vi "Read_configuration.vi"(8 "error in (no error)":errorcluster, 11 "configuration file path":path) -> (0 "error out":errorcluster, 3 "output cluster":T1)   [LabVIEW 2015]
uses:
  <vilib>/LabVIEW Targets/FPGA/cRIO/shared/nicrio_ModuleControls/nicrio_cRIO-9234_DataRatesRing2.ctl
  <vilib>/Utility/config.llb/Read Key (Double).vi
  <vilib>/Utility/config.llb/Read Key (String).vi
  <vilib>/Utility/config.llb/Read Key (U32).vi
  <vilib>/Utility/config.llb/Read Key (Boolean).vi
  <vilib>/Utility/config.llb/NI_LVConfig.lvlib
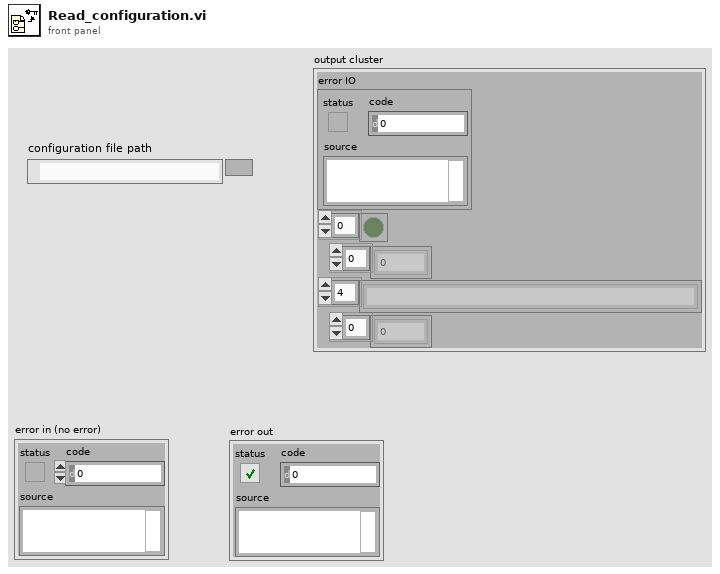
[diagram p1: front panel]
types:
  T1 = cluster{"error IO":errorcluster, bool[], u32[], string[], dbl[]}
  T2 = typedef "nicrio_cRIO-9234_DataRatesRing2.ctl" = u8
  T3 = typedef "NI_LVConfig.lvlib/Config Data RefNum.ctl" = refnum<k1>
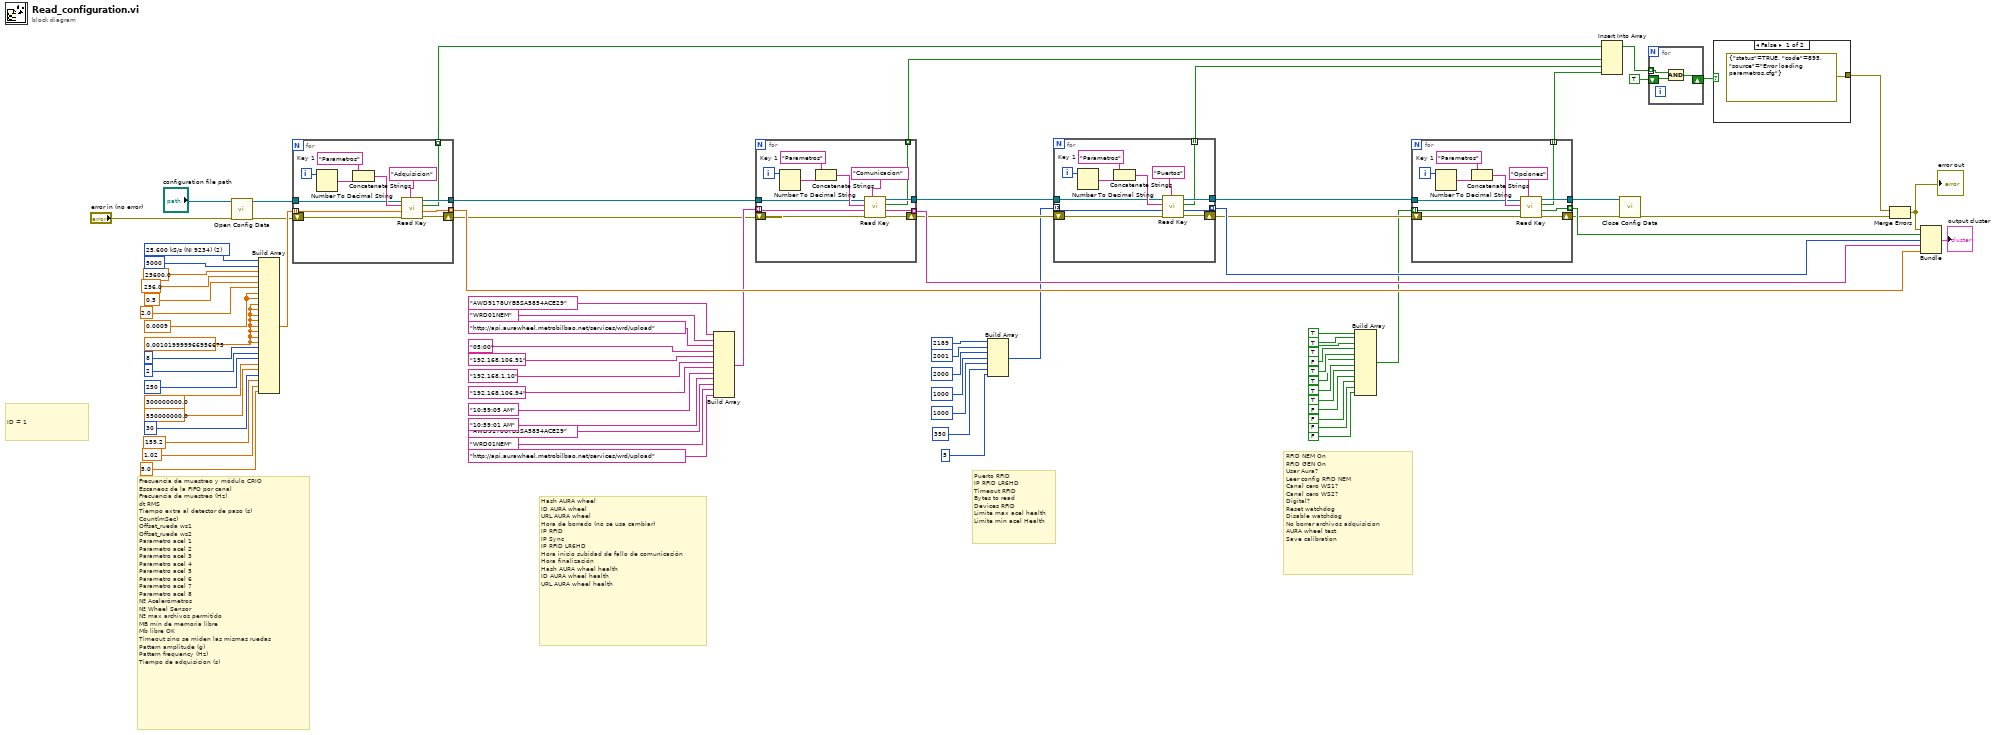
[diagram p0: block diagram]
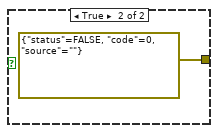
[diagram p2: hidden frame]
diagram:
  w34 = T2 2 items=["51.200 kS/s (NI 9234)"=1, "25.600 kS/s (NI 9234)"=2, "17.067 kS/s (NI 9234)"=3, "12.800 kS/s (NI 9234)"=4, "10.240 kS/s (NI 9234)"=5, "8.533 kS/s (NI 9234)"=6, "7.314 kS/s (NI 9234)"=7, "6.400 kS/s (NI 9234)"=8, "5.689 kS/s (NI 9234)"=9, "5.120 kS/s (NI 9234)"=10, "4.654 kS/s (NI 9234)"=11, "4.267 kS/s (NI 9234)"=12, "3.938 kS/s (NI 9234)"=13, "3.657 kS/s (NI 9234)"=14, "3.413 kS/s (NI 9234)"=15, "3.200 kS/s (NI 9234)"=16, "3.012 kS/s (NI 9234)"=17, "2.845 kS/s (NI 9234)"=18, "2.695 kS/s (NI 9234)"=19, "2.560 kS/s (NI 9234)"=20, "2.438 kS/s (NI 9234)"=21, "2.328 kS/s (NI 9234)"=22, "2.226 kS/s (NI 9234)"=23, "2.133 kS/s (NI 9234)"=24, "2.048 kS/s (NI 9234)"=25, "1.969 kS/s (NI 9234)"=26, "1.896 kS/s (NI 9234)"=27, "1.829 kS/s (NI 9234)"=28, "1.765 kS/s (NI 9234)"=29, "1.707 kS/s (NI 9234)"=30, "1.652 kS/s (NI 9234)"=31] ("Data Rate")
  w15 = 0.0009 ("element")
  w33 = sgl 0.00102
  # "RFID NEM On\nRFID GEN On\nUsar Aura?\nLeer config RFID NEM\nCanal cero WS1?\nCanal cero WS2?\nDigital?\nReset watchdog\nDisable watchdog\nNo borrar archivos adquisicion\nAURA wheel test\nSave calibration"
  # "Puerto RFID\nIP RFID LR6HD\nTimeout RFID\nBytes to read\nDevices RFID\nLimite max acel health\nLimite min acel Health"
  # "Hash AURA wheel\nID AURA wheel\nURL AURA wheel\nHora de borrado (no se usa cambiar)\nIP RFID\nIP Sync\nIP RFID LR6HD\nHora inicio subidad de fallo de comunicación\nHora finalización\nHash AURA wheel health\nID AURA wheel health\nURL AURA wheel health"
  # "Frecuencia de muestreo y módulo CRIO\nEscaneos de la FIFO por canal\nFrecuencia de muestreo (Hz)\ndt RMS\nTiempo extra al detector de paso (s)\nCount(mSec)\nOffset_rueda ws1\nOffset_rueda ws2\nParametro acel 1\nParametro acel 2\nParametro acel 3\nParametro acel 4\nParametro acel 5\nParametro acel 6\nParametro acel 7\nParametro acel 8\nNº Acelerómetros\nNº Wheel Sensor\nNº max archivos permitido\nMB mín de memoria libre\nMb libre OK\nTimeout sino se miden las mismas ruedas\nPattern amplitude (g)\nPattern frequency (Hz)\nTiempo de adquisicion (s)"
  # "ID = 1"
  n1 = call <vilib>:"Open Config Data.vi"("error in (no error)"="error in (no error)", "configuration file path"="configuration file path") -> ("error out"=w51:errorcluster, "refnum"=w52:T3)  [unwired: 1 in, 7 out]
  n2 = Build Array(w34, 5000, 25600.0 ("element"), 256.0 ("element"), 0.5 ("element"), 2.0 ("element"), w15, w15, w33, w33, w33, w33, w33, w33, w33, w33, 8, 2, 250, 300000000.0, 550000000.0, 30, 159.2, 1.02, 5.0) -> (w61:dbl[])
  n3 = for {
    tunnel: w52 -> [w86]
    shift-right: [w84] -> w47
    shift-left: w51 -> [w85]
    tunnel: [w83] -> w48
    tunnel: [w82] -> w79 mode=indexing
    tunnel: [w81] -> w50 mode=indexing
    tunnel: w61 -> [w80] mode=indexing
    i -> [w90]
    w88 = "Parametros"  # Key 1
    n4 = Number To Decimal String(number=w90) -> (decimal integer string=w89:string)  [unwired: 1 in]
    n5 = Concatenate Strings(w88, w89) -> (w87:string)
    n6 = call-poly <vilib>:"Read Key.vi"("section"="Adquisicion", "error in (no error)"=w85, "default value"=w80, "key"=w87, "refnum"=w86) -> ("error out"=w84:errorcluster, "value"=w82:dbl, "found?"=w81:bool, "refnum out"=w83:T3)  [unwired: 3 in]
  }
  n7 = Build Array("AWD9178UYB5SA5854ACE29" ("URL LOGIN"), "WRD01NEM" ("URL ENVÍO PARAM"), "http://api.aurawheel.metrobilbao.net/services/wrd/upload" ("URL LOGOUT"), "05:00", "192.168.106.91" ("element"), "192.168.1.10" ("Time Server\nIP Address"), "192.168.106.94" ("Time Server\nIP Address"), "10:59:05 AM" ("element"), "10:59:01 AM" ("element"), "AWD9178UYB5SA5854ACE29" ("URL LOGIN"), "WRD01NEM" ("URL ENVÍO PARAM"), "http://api.aurawheel.metrobilbao.net/services/wrd/upload" ("URL LOGOUT")) -> (w60:string[])
  n8 = for {
    tunnel: w48 -> [w98]
    shift-right: [w96] -> w70
    shift-left: w47 -> [w97]
    tunnel: [w95] -> w69
    tunnel: [w94] -> w78 mode=indexing
    tunnel: [w93] -> w46 mode=indexing
    tunnel: w60 -> [w92] mode=indexing
    i -> [w102]
    w100 = "Parametros"  # Key 1
    n9 = Number To Decimal String(number=w102) -> (decimal integer string=w101:string)  [unwired: 1 in]
    n10 = Concatenate Strings(w100, w101) -> (w99:string)
    n11 = call-poly <vilib>:"Read Key.vi"("section"="Comunicacion", "error in (no error)"=w97, "default value"=w92, "key"=w99, "refnum"=w98) -> ("error out"=w96:errorcluster, "value"=w94:string, "found?"=w93:bool, "refnum out"=w95:T3)  [unwired: 3 in]
  }
  n12 = Build Array(u16 2189 ("element"), u16 2001 ("element"), u16 2000 ("element"), u16 1000 ("element"), u16 1000 ("element"), u16 350 ("element"), u16 5 ("element")) -> (w59:u16[])
  n13 = for {
    tunnel: w69 -> [w110]
    shift-right: [w108] -> w72
    shift-left: w70 -> [w109]
    tunnel: [w107] -> w71
    tunnel: [w106] -> w77 mode=indexing
    tunnel: [w105] -> w45 mode=indexing
    tunnel: w59 -> [w104] mode=indexing
    i -> [w114]
    w112 = "Parametros"  # Key 1
    n14 = Number To Decimal String(number=w114) -> (decimal integer string=w113:string)  [unwired: 1 in]
    n15 = Concatenate Strings(w112, w113) -> (w111:string)
    n16 = call-poly <vilib>:"Read Key.vi"("section"="Puertos", "error in (no error)"=w109, "default value"=w104, "key"=w111, "refnum"=w110) -> ("error out"=w108:errorcluster, "value"=w106:u32, "found?"=w105:bool, "refnum out"=w107:T3)  [unwired: 3 in]
  }
  n17 = Build Array(TRUE, TRUE, TRUE, FALSE ("element"), TRUE ("element"), TRUE ("element"), TRUE ("element"), TRUE ("element"), FALSE ("element"), FALSE ("element"), FALSE ("element"), FALSE ("element")) -> (w56:bool[])
  n18 = for {
    tunnel: w71 -> [w122]
    shift-right: [w120] -> w73
    shift-left: w72 -> [w121]
    tunnel: [w119] -> w74
    tunnel: [w118] -> w76 mode=indexing
    tunnel: [w117] -> w44 mode=indexing
    tunnel: w56 -> [w116] mode=indexing
    i -> [w126]
    w124 = "Parametros"  # Key 1
    n19 = Number To Decimal String(number=w126) -> (decimal integer string=w125:string)  [unwired: 1 in]
    n20 = Concatenate Strings(w124, w125) -> (w123:string)
    n21 = call-poly <vilib>:"Read Key.vi"("section"="Opciones", "error in (no error)"=w121, "default value"=w116, "key"=w123, "refnum"=w122) -> ("error out"=w120:errorcluster, "value"=w118:bool, "found?"=w117:bool, "refnum out"=w119:T3)  [unwired: 3 in]
  }
  n22 = Insert Into Array(array=w50, new element #1=w46, new element #2=w45, new element #3=w44) -> (w53:bool[])  [unwired: 1 in]
  n23 = call <vilib>:"Close Config Data.vi"("error in (no error)"=w73, "refnum"=w74) -> ("error out"=w67:errorcluster)  [unwired: 8 in, 1 out]
  n24 = for {
    shift-right: [w129] -> w54
    shift-left: TRUE -> [w130]
    tunnel: w53 -> [w128] mode=indexing
    n25 = Compound Arithmetic op=AND(w128, w130) -> (w129:bool)
  }
  n26 = case shown="False" w54 {
    tunnel: [errorcluster {"status"=TRUE, "code"=895, "source"="Error loading parametros.cfg"} ("error out") errorcluster {"status"=FALSE, "code"=0, "source"=""} ("error out")] -> w68
    frame False {
    }
    frame True {
    }
  }
  n27 = Merge Errors(w68, w67) -> (w66:errorcluster)
  "error out" <- w66
  n28 = Bundle("error IO"=w66, w76, w77, w78, w79) -> (→"output cluster":T1)  [unwired: 1 in]
